vi "set images.vi"(8 "error in (no error)":errorcluster caption="Fehler (Eingang, kein Fehler)", 10 "images":refnum<class "img.lvclass">[](array[class]), 11 "Setup (Eingang)":refnum<class "Setup.lvclass">) -> (0 "error out":errorcluster caption="Fehler (Ausgang)", 3 "Setup (Ausgang)":refnum<class "Setup.lvclass">)   [LabVIEW 2013, in "DatenKlassen.lvlib" / "Setup.lvclass"]
uses:
  Setup.lvclass
  Image/img.lvclass
  Setup.lvclass/Setup.ctl
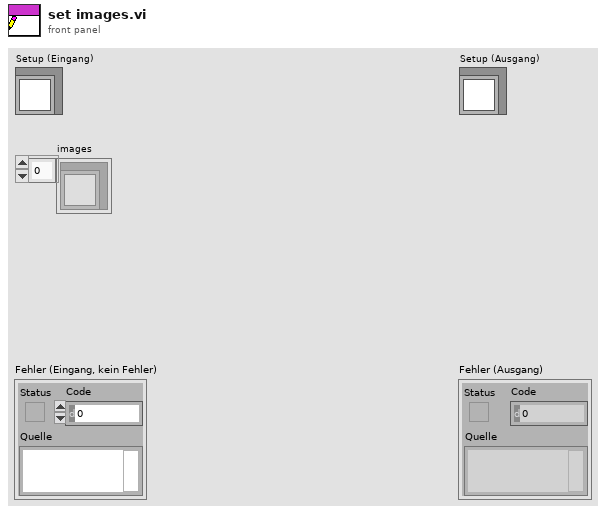
[diagram p1: front panel]
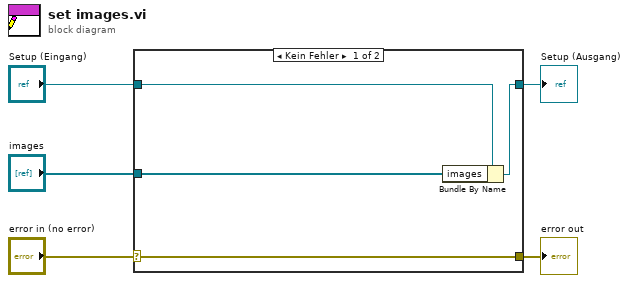
[diagram p0: block diagram]
diagram:
  n1 = case shown="Kein Fehler" "error in (no error)" {
    selector: "error in (no error)" -> [w9 w10]
    tunnel: [w9 w10] -> w4
    tunnel: [w7 w11] -> w2
    tunnel: "Setup (Eingang)" -> [w8 w11]
    tunnel: "images" -> [w6 _]
    frame No Error {
      n2 = Bundle By Name(cluster=w8, "images"=w6) -> (w7:refnum<class "Setup.lvclass">)
    }
    frame Error {
    }
  }
  "error out" <- w4
  "Setup (Ausgang)" <- w2
